vi "initialize_Host.vi"(5 "error in (no error)":errorcluster) -> (14 "MoAgSy_Host out":refnum<class "MoAgSy_Host.lvclass">, 16 "Canceled":bool, 19 "error out":errorcluster)   [LabVIEW 2009, in "MoAgSy.lvlib" / "MoAgSy_Host.lvclass"]
doc: "<B>public</B> VI initializes Host.\nReads init file. If no success, tries to create new Host.\nIf cancelled, Host out is emty labview object. To more specific class will provide an error!\n\nF.Berck@gsi.de\nGSI Darmstadt 2009"
uses:
  MoAgSy_Host.lvclass
  MoAgSy_Host.lvclass/MoAgSy_Host.ctl
  MoAgSy.lvlib
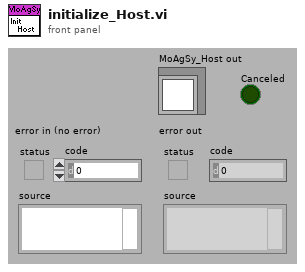
[diagram p1: front panel]
types:
  T1 = cluster{"Working Folder":path, "Class Folder":path}
  T2 = cluster{"FTP Host":string, "FTP Username":string, "FTP Password":string, "remote port (21)":u16, "Load new libs from FTP Server":bool}
  T3 = cluster{"Host Name":string, "Maximum number of running Agents":i16, "ID":string}
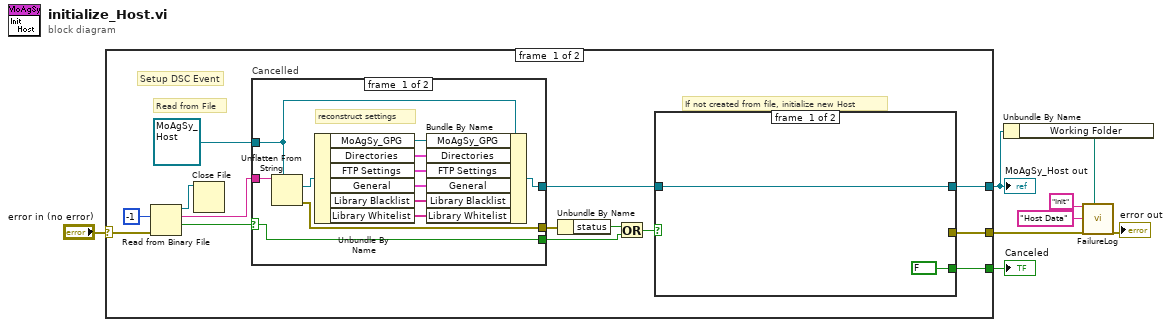
[diagram p0: block diagram]
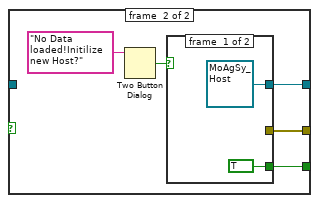
[diagram p2: hidden frame]
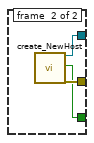
[diagram p3: hidden frame]
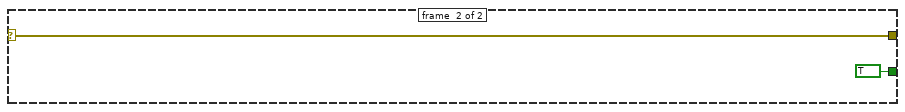
[diagram p5: hidden frame]
diagram:
  n1 = case shown="No Error" "error in (no error)" {
    selector: "error in (no error)" -> [w20 w50]
    tunnel: [w10 w50] -> w2
    tunnel: [w12 _] -> w6
    tunnel: [w9 TRUE ("Cancel")] -> w7
    frame #0 {
      # "Setup DSC Event"
      # "If not created from file, initialize new Host"
      # "Read from File"
      n2 = Read from Binary File(8:w20, 10:-1 ("count (1)")) -> (1:w19:bool, 2:w22:string, 3:w18:refnum<file>)  [unwired: 5 out]
      n3 = Close File(refnum=w18) -> ()  [unwired: 1 in, 2 out]
      n4 = case "Cancelled" shown="False" w19 {
        selector: w19 -> [w38 w47]
        tunnel: w22 -> [w46 _]
        tunnel: [w45 w48] -> w13
        tunnel: refnum<class "MoAgSy_Host.lvclass"> refnum ("MoAgSy.lvlib:MoAgSy_Host.lvclass") -> [w42 w48]
        tunnel: [w40 _] -> w11
        tunnel: [w38 w47] -> w14
        frame #0 {
          # "reconstruct settings"
          n5 = Unflatten From String(type=w42, binary string=w46) -> (value=w41:refnum<class "MoAgSy_Host.lvclass">, error out=w40:errorcluster)  [unwired: 1 in, 3 out]
          n6 = Unbundle By Name(w41) -> ("MoAgSy_GPG"=w35:refnum<class "MoAgSy_GPG.lvclass">, "Directories"=w44:T1, "FTP Settings"=w43:T2, "General"=w39:T3, "Library Blacklist"=w36:string[], "Library Whitelist"=w37:string[])
          n7 = Bundle By Name(cluster=w42, "MoAgSy_GPG"=w35, "Directories"=w44, "FTP Settings"=w43, "General"=w39, "Library Blacklist"=w36, "Library Whitelist"=w37) -> (w45:refnum<class "MoAgSy_Host.lvclass">)
        }
        frame #1 {
        }
      }
      n8 = Unbundle By Name(w11) -> ("status"=w15:bool)
      n9 = Or(x=w15, y=w14) -> (x .or. y?=w16:bool)
      n10 = case shown="True" w16 {
        tunnel: w13 -> [w24 _]
        tunnel: [w24 w29] -> w12
        tunnel: [_ w28] -> w10
        tunnel: [FALSE ("Cancel") w27] -> w9
        frame #0 {
        }
        frame #1 {
          n11 = Two Button Dialog(message="No Data loaded!Initilize new Host?") -> (T button?=w25:bool)  [unwired: 2 out]
          n12 = case shown="True" w25 {
            tunnel: [refnum<class "MoAgSy_Host.lvclass"> refnum ("MoAgSy_Host.lvclass out") w34] -> w29
            tunnel: [_ w33] -> w28
            tunnel: [TRUE ("Cancel") w32] -> w27
            frame #0 {
            }
            frame #1 {
              n13 = call "create_NewHost.vi"() -> ("MoAgSy_Host.lvclass out"=w34:refnum<class "MoAgSy_Host.lvclass">, "Cancel"=w32:bool, "error out"=w33:errorcluster)  [unwired: 17 out]
            }
          }
        }
      }
    }
    frame #1 {
    }
  }
  "MoAgSy_Host out" <- w6
  "Canceled" <- w7
  n14 = Unbundle By Name(w6) -> ("Working Folder"=w5:path)
  n15 = call "FailureLog.vi"("Section"="Init", "key"="Host Data", "error in (no error)"=w2, "Path"=w5) -> ("error out"=→"error out":errorcluster)  [unwired: 15 in]
